vi "H5Pget_fapl_family.vi"(6 "error in (no error)":errorcluster, 9 "HDF5 Property List Ref":T1) -> (0 "error out":errorcluster, 1 "Member File Access Property List ID":T1, 2 "Member Size":u64, 3 "HDF5 Property List Ref out":T1)   [LabVIEW 2017]
doc: "Returns file access property list information."
uses:
  <vilib>/UPVI/lvhdf5/library.llb/HDF5 Ref.ctl
  <vilib>/UPVI/lvhdf5/hdf5.dll
panel:
  # "LVHDF5 Toolkit\nCopyright (c) 2005-2013 by Jason D. Sommerville\nCopyright (c) 2014 by UPVI, LLC.\n\nThis use and distribution of this file is governed by the terms found in \nLICENSE.txt distributed with this toolkit and installed at\n <user.lib>\\_lvhdf5\\LICENSE.txt"
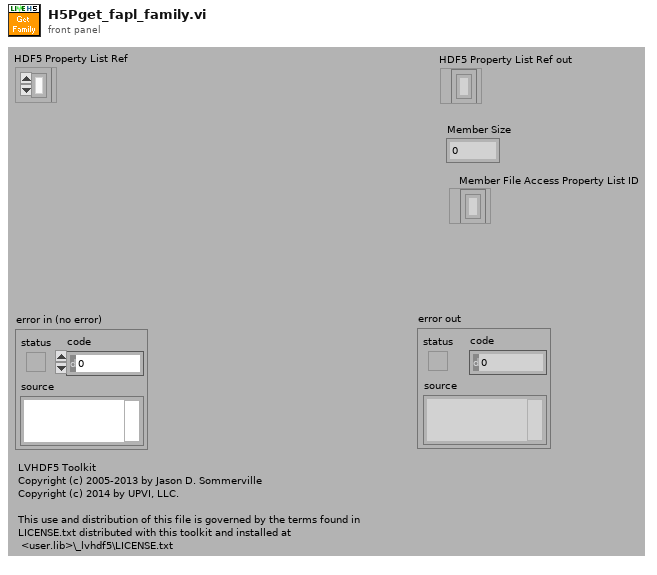
[diagram p1: front panel]
types:
  T1 = typedef "HDF5 Ref.ctl" = refnum<k1>
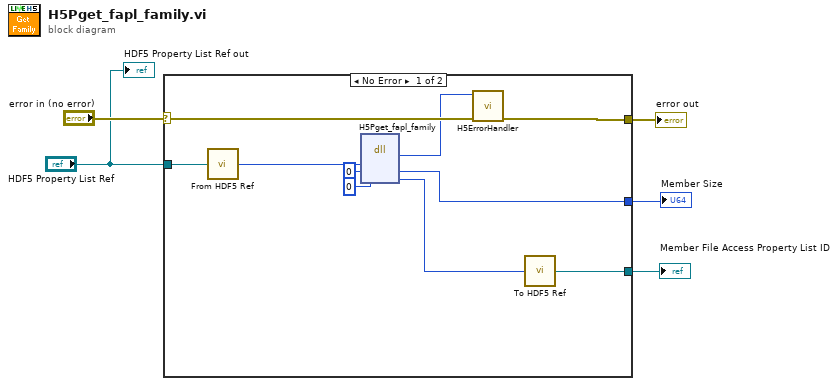
[diagram p0: block diagram]
diagram:
  n1 = case shown="No Error" "error in (no error)" {
    selector: "error in (no error)" -> [w15 w16]
    tunnel: [w6 w16] -> w4
    tunnel: "HDF5 Property List Ref" -> [w14 _]
    tunnel: [w7 _] -> w2
    tunnel: [w8 _] -> w1
    frame No Error {
      n2 = call <vilib>:"From HDF5 Ref.vi"("HDF5 Ref"=w14) -> ("I32"=w13:i32)
      n3 = dll-call lib="C:/Program Files/National Instruments/LabVIEW 2017/vi.lib/UPVI/lvhdf5/hdf5.dll" fn="H5Pget_fapl_family"("plist_id"=w13, "memb_size"=u64 0, "memb_fapl_id"=0) -> ("return type"=w12:i32, "memb_size"=w7:u64, "memb_fapl_id"=w9:i32)  [unwired: 4 in, 2 out]
      n4 = call <vilib>:"H5ErrorHandler.vi"("error in (no error)"=w15, "herr_t"=w12) -> ("error out"=w6:errorcluster)  [unwired: 3 in, 4 out]
      n5 = call <vilib>:"To HDF5 Ref.vi"("I32"=w9) -> ("HDF5 Ref"=w8:T1)
    }
    frame Error {
    }
  }
  "error out" <- w4
  "Member Size" <- w2
  "Member File Access Property List ID" <- w1
  "HDF5 Property List Ref out" <- "HDF5 Property List Ref"
